vi "创建隐藏文件夹.vi"   [LabVIEW 2018]
uses:
  <vilib>/Utility/error.llb/DialogType.ctl
types:
  T1 = typedef "DialogType.ctl" = u16
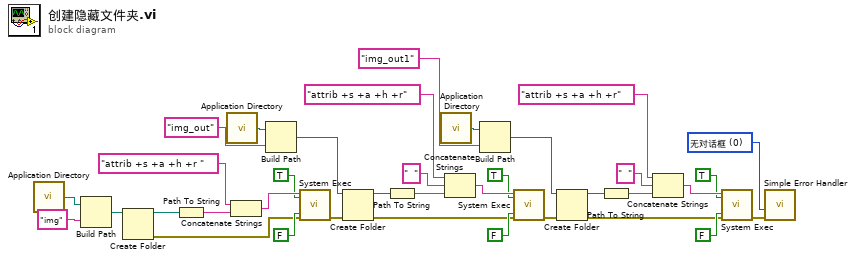
[diagram p0: block diagram]
diagram:
  w19 = T1 0 items=["无对话框", "确定信息", "继续或停止信息", "确定信息＋警告", "继续/停止+警告"] ("type of dialog (OK msg:1)")
  n1 = call <vilib>:"Application Directory.vi"() -> ("Application Directory"=w36:path)
  n2 = Build Path(base path=w36, name or relative path="img" ("名称或相对路径")) -> (appended path=w35:path)
  n3 = Create Folder(path (use dialog)=w35) -> (created path=w32:path, error out=w1:errorcluster)  [unwired: 2 in, 1 out]
  n4 = Path To String(path=w32) -> (string=w13:string)
  n5 = call <vilib>:"Application Directory.vi"() -> ("Application Directory"=w23:path)
  n6 = Concatenate Strings("attrib +s +a +h +r " ("字符串"), w13) -> (w31:string)
  n7 = Build Path(base path=w23, name or relative path="img_out" ("名称或相对路径")) -> (appended path=w24:path)
  n8 = call <vilib>:"System Exec.vi"("run minimized? (F)"=FALSE, "wait until completion? (T)"=TRUE, "error in (no error)"=w1, "command line"=w31) -> ("error out"=w2:errorcluster)  [unwired: 4 in, 3 out]
  n9 = Create Folder(path (use dialog)=w24, error in=w2) -> (created path=w28:path, error out=w3:errorcluster)  [unwired: 1 in, 1 out]
  n10 = Path To String(path=w28) -> (string=w29:string)
  n11 = call <vilib>:"Application Directory.vi"() -> ("Application Directory"=w22:path)
  n12 = Concatenate Strings("attrib +s +a +h +r" ("字符串"), "  " ("字符串"), w29) -> (w30:string)
  n13 = Build Path(base path=w22, name or relative path="img_out1" ("名称或相对路径")) -> (appended path=w21:path)
  n14 = call <vilib>:"System Exec.vi"("run minimized? (F)"=FALSE, "wait until completion? (T)"=TRUE, "error in (no error)"=w3, "command line"=w30) -> ("error out"=w4:errorcluster)  [unwired: 4 in, 3 out]
  n15 = Create Folder(path (use dialog)=w21, error in=w4) -> (created path=w16:path, error out=w5:errorcluster)  [unwired: 1 in, 1 out]
  n16 = Path To String(path=w16) -> (string=w15:string)
  n17 = Concatenate Strings("attrib +s +a +h +r" ("字符串"), "  " ("字符串"), w15) -> (w14:string)
  n18 = call <vilib>:"System Exec.vi"("run minimized? (F)"=FALSE, "wait until completion? (T)"=TRUE, "error in (no error)"=w5, "command line"=w14) -> ("error out"=w6:errorcluster)  [unwired: 4 in, 3 out]
  n19 = call <vilib>:"Simple Error Handler.vi"("type of dialog (OK msg:1)"=w19, "error in (no error)"=w6) -> ()  [unwired: 3 in, 5 out]
